vi "WaitFor.vi"(4 "Wait For Chamber":bool, 5 "Timeout":dbl, 6 "Wait For Position":bool, 7 "Delay":dbl, 8 "Wait For Field":bool, 9 "Wait For Temperature":bool, 10 "error in (no error)":errorcluster, 11 "Instrument Ref In":refnum<k24>) -> (2 "error out":errorcluster, 3 "Instrument Ref Out":refnum<k24>)   [LabVIEW 2016]
uses:
  C:/user/patrick/hg/levylab_inst_ppms2/lvsrc/PPMS2/QDInstrument_LabView/QDInstrument.dll
  QDInstrument.dll
  Instance           2 15Saved   WaitFor .vi
  Instance           1 15Saved   WaitFor .vi
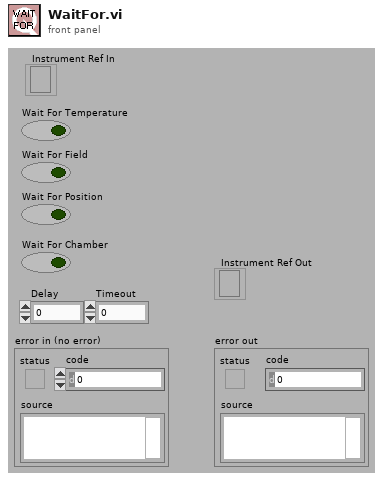
[diagram p1: front panel]
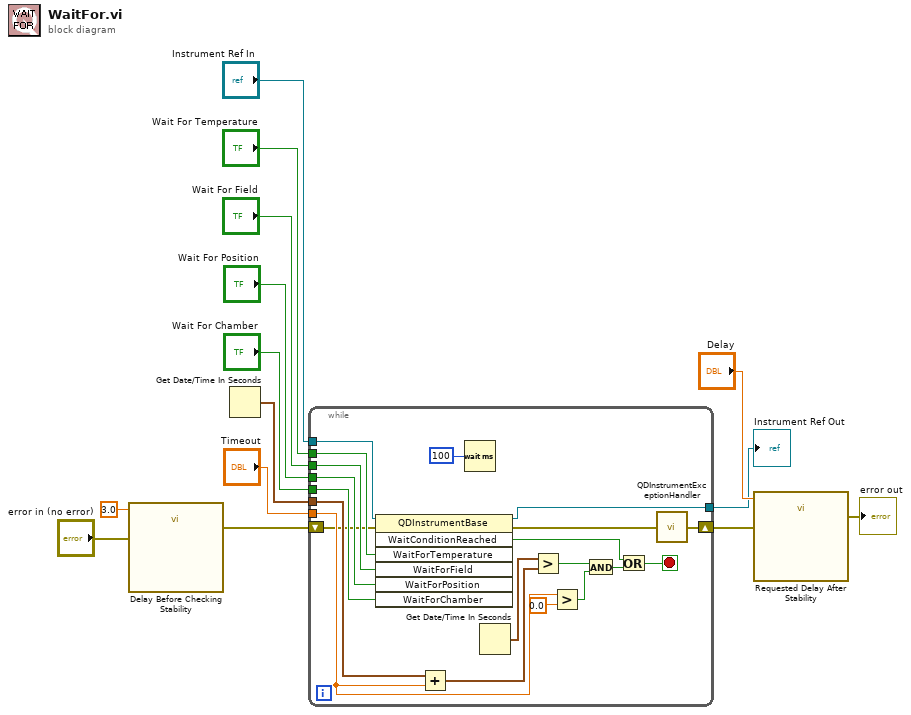
[diagram p0: block diagram]
diagram:
  n1 = call "Delay Before Checking Stability"("error in (no error)"="error in (no error)", "Delay Time (s)"=3.0) -> ("error out"=w5:errorcluster)  [unwired: 9 in]
  n2 = Get Date/Time In Seconds() -> (seconds since 1Jan1904=w4:timestamp)
  n3 = while {
    shift-right: [w15] -> w10
    shift-left: w5 -> [w18]
    tunnel: "Wait For Temperature" -> [w22]
    tunnel: "Wait For Field" -> [w21]
    tunnel: "Wait For Position" -> [w20]
    tunnel: "Wait For Chamber" -> [w19]
    tunnel: w4 -> [w33]
    tunnel: "Timeout" -> [w30]
    tunnel: "Instrument Ref In" -> [w24]
    tunnel: [w23] -> w1
    stop <- w25 stop-if-true
    n4 = invoke class="QDInstrumentBase" method="WaitConditionReached"(reference=w24, error in=w18, "WaitForTemperature"=w22, "WaitForField"=w21, "WaitForPosition"=w20, "WaitForChamber"=w19) -> (reference out=w23:refnum<k24>, error out=w16:errorcluster, "WaitConditionReached"=w17:bool)  [unwired: 1 in, 4 out]
    n5 = Add(x=w33, y=w30) -> (x+y=w31:timestamp)
    n6 = Wait (ms)(milliseconds to wait=u32 100) -> ()  [unwired: 1 out]
    n7 = Get Date/Time In Seconds() -> (seconds since 1Jan1904=w32:timestamp)
    n8 = Greater?(x=w32, y=w31) -> (0:w28:bool)
    n9 = Greater?(x=w30, y=0.0) -> (0:w27:bool)
    n10 = And(x=w28, y=w27) -> (x .and. y?=w26:bool)
    n11 = Or(x=w17, y=w26) -> (x .or. y?=w25:bool)
    n12 = call "QDInstrumentExceptionHandler.vi"("Error in"=w16) -> ("Error out"=w15:errorcluster)
  }
  "Instrument Ref Out" <- w1
  n13 = call "Requested Delay After Stability"("error in (no error)"=w10, "Delay Time (s)"="Delay") -> ("error out"=→"error out":errorcluster)  [unwired: 9 in]
